vi "Seconds to HMS.vi"(1 "Time Elapsed in Seconds":dbl) -> (0 "Time Elapsed (H : M : S)":string)   [LabVIEW 2013]
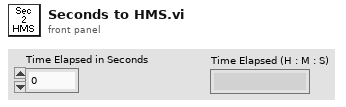
[diagram p1: front panel]
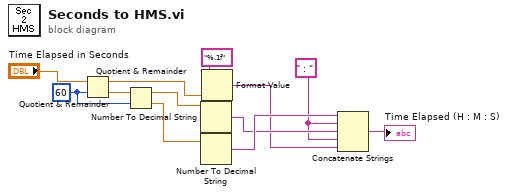
[diagram p0: block diagram]
diagram:
  w5 = " : "
  w10 = 60 ("y")
  n1 = Quotient & Remainder(x="Time Elapsed in Seconds", y=w10) -> (x-y*floor(x/y)=w2:dbl, floor(x/y)=w11:dbl)
  n2 = Quotient & Remainder(x=w11, y=w10) -> (x-y*floor(x/y)=w9:dbl, floor(x/y)=w8:dbl)
  n3 = Number To Decimal String(number=w9) -> (decimal integer string=w6:string)  [unwired: 1 in]
  n4 = Number To Decimal String(number=w8) -> (decimal integer string=w7:string)  [unwired: 1 in]
  n5 = Format Value(format string="%.1f", value (0)=w2) -> (output string=w1:string)  [unwired: 1 in]
  n6 = Concatenate Strings(w7, w5, w6, w5, w1) -> (→"Time Elapsed (H : M : S)":string)
